vi "Peregrine_set_position.vi"(0 "Handle in":refnum<visa-resource-name>, 2 "Address":u8, 7 "New position":i32, 11 "error":errorcluster) -> (4 "Handle out":refnum<visa-resource-name>, 6 "Key response":u32, 8 "Value response":i32, 15 "error out":errorcluster)   [LabVIEW 2019]
panel:
  out "Command":i32
  out "Address response":u8
  # "Inputs"
  # "Response message"
  # "Output"
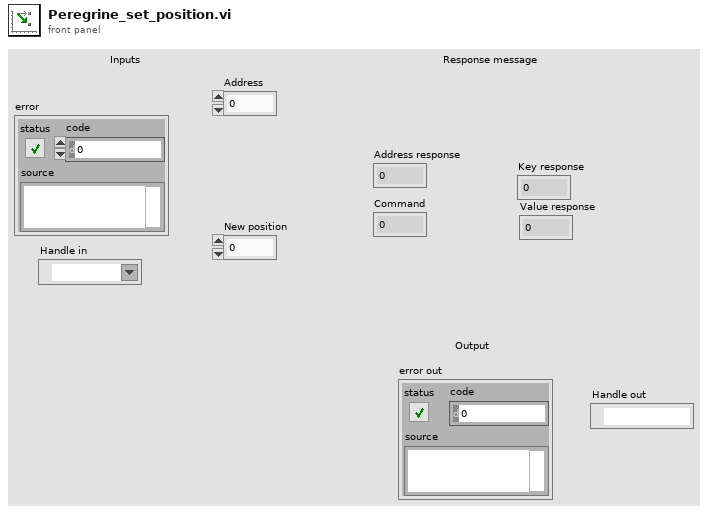
[diagram p1: front panel]
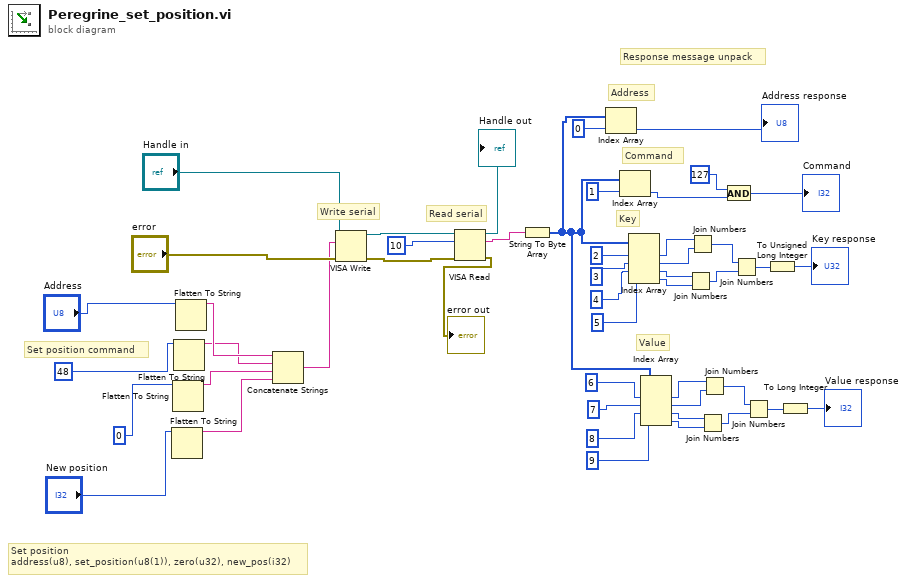
[diagram p0: block diagram]
diagram:
  # "Value"
  # "Response message unpack"
  # "Set position command"
  # "Command"
  # "Address"
  # "Key"
  # "Read serial"
  # "Write serial"
  # "Set position\naddress(u8), set_position(u8(1)), zero(u32), new_pos(i32)"
  n1 = Flatten To String(anything="New position") -> (data string=w21:string)  [unwired: 3 in, 2 out]
  n2 = Flatten To String(anything=0) -> (data string=w22:string)  [unwired: 3 in, 2 out]
  n3 = Flatten To String(anything=u8 48) -> (data string=w23:string)  [unwired: 3 in, 2 out]
  n4 = Flatten To String(anything="Address") -> (data string=w25:string)  [unwired: 3 in, 2 out]
  n5 = Concatenate Strings(w25, w23, w22, w21) -> (w20:string)
  n6 = VISA Write(VISA resource name="Handle in", write buffer=w20, error in (no error)="error") -> (VISA resource name out=w48:refnum<visa-resource-name>, error out=w27:errorcluster)  [unwired: 1 out]
  n7 = VISA Read(VISA resource name=w48, byte count=10, error in (no error)=w27) -> (VISA resource name out=→"Handle out":refnum<visa-resource-name>, read buffer=w46:string, error out=→"error out":errorcluster)  [unwired: 1 out]
  n8 = String To Byte Array(string=w46) -> (unsigned byte array=w11:u8[])
  n9 = Index Array(array=w11, index=0) -> (element=→"Address response":u8)
  n10 = Index Array(array=w11, index=1) -> (element=w3:u8)
  n11 = Index Array(array=w11, index #1=2, index #2=3, index #3=4, index #4=5) -> (element #1=w39:u8, element #2=w38:u8, element #3=w37:u8, element #4=w36:u8)
  n12 = Index Array(array=w11, index #1=6, index #2=7, index #3=8, index #4=9) -> (element #1=w18:u8, element #2=w17:u8, element #3=w16:u8, element #4=w15:u8)
  n13 = Join Numbers(hi=w37, lo=w36) -> ((hi.lo)=w35:u16)
  n14 = Join Numbers(hi=w39, lo=w38) -> ((hi.lo)=w34:u16)
  n15 = Join Numbers(hi=w16, lo=w15) -> ((hi.lo)=w14:u16)
  n16 = Join Numbers(hi=w18, lo=w17) -> ((hi.lo)=w13:u16)
  n17 = And(x=127, y=w3) -> (x .and. y?=→"Command":i32)
  n18 = Join Numbers(hi=w34, lo=w35) -> ((hi.lo)=w6:u32)
  n19 = Join Numbers(hi=w13, lo=w14) -> ((hi.lo)=w7:u32)
  n20 = To Unsigned Long Integer(number=w6) -> (unsigned 32bit integer=→"Key response":u32)
  n21 = To Long Integer(number=w7) -> (32bit integer=→"Value response":i32)
